vi "Inspect Address Pads.vi"(7 "Console Log in":refnum<class "Console Log.lvclass">, 8 "error in":errorcluster, 10 "Module Data In":T1={"TBM-TBM"={"Fiducial Image"={"Image Position"=refnum, "Image Reference"=refnum, "Field of View"={"x(mm)"=0.0, "y(mm)"=0.0}}, "Fiducials"=[]}, "TBM-HDI"={"Fiducial Image"={"Image Position"=refnum, "Image Reference"=refnum, "Field of View"={"x(mm)"=0.0, "y(mm)"=0.0}}, "Fiducials"=[]}, "Address Pads"={"Fiducial Image"={"Image Position"=refnum, "Image Reference"=refnum, "Field of View"={"x(mm)"=0.0, "y(mm)"=0.0}}, "Fiducials"=[]}, "HDI Bond Pad References"=[], "BBM Bond Pad References"=[], "HV-HDI"={"Fiducial Image"={"Image Position"=refnum, "Image Reference"=refnum, "Field of View"={"x(mm)"=0.0, "y(mm)"=0.0}}, "Selected Fiducial"={"Fiducial Image Coordinate"=refnum, "Fiducial Source"=enum."Pattern Recognition"}, "fiducial name"=""}, "HV-BBM"={"Fiducial Image"={"Image Position"=refnum, "Image Reference"=refnum, "Field of View"={"x(mm)"=0.0, "y(mm)"=0.0}}, "Selected Fiducial"={"Fiducial Image Coordinate"=refnum, "Fiducial Source"=enum."Pattern Recognition"}, "fiducial name"=""}, "Chuck"=0, "Slot"=0, "Potting Selection"={"HDI Bond Pads"=[TRUE, TRUE, TRUE, TRUE, TRUE, TRUE, TRUE, TRUE, TRUE, TRUE, TRUE, TRUE, TRUE, TRUE, TRUE, TRUE], "BBM Bond Pads"=[TRUE, TRUE, TRUE, TRUE, TRUE, TRUE, TRUE, TRUE, TRUE, TRUE, TRUE, TRUE, TRUE, TRUE, TRUE, TRUE], "TBM Inner"={"Top"=TRUE, "Left"=TRUE, "Bottom"=TRUE, "Right"=TRUE}, "TBM Outer"={"Top"=TRUE, "Left"=TRUE, "Bottom"=TRUE, "Right"=TRUE}, "Address Pads"={"Top"=TRUE, "Bottom"=TRUE}, "High Voltage"={"HDI"=TRUE, "BBM"=TRUE}}}, 11 "Potting Procedure in":refnum<class "Potting Procedure.lvclass">) -> (0 "error out":errorcluster, 2 "Module Data Out":T1={"TBM-TBM"={"Fiducial Image"={"Image Position"=refnum, "Image Reference"=refnum, "Field of View"={"x(mm)"=0.0, "y(mm)"=0.0}}, "Fiducials"=[]}, "TBM-HDI"={"Fiducial Image"={"Image Position"=refnum, "Image Reference"=refnum, "Field of View"={"x(mm)"=0.0, "y(mm)"=0.0}}, "Fiducials"=[]}, "Address Pads"={"Fiducial Image"={"Image Position"=refnum, "Image Reference"=refnum, "Field of View"={"x(mm)"=0.0, "y(mm)"=0.0}}, "Fiducials"=[]}, "HDI Bond Pad References"=[], "BBM Bond Pad References"=[], "HV-HDI"={"Fiducial Image"={"Image Position"=refnum, "Image Reference"=refnum, "Field of View"={"x(mm)"=0.0, "y(mm)"=0.0}}, "Selected Fiducial"={"Fiducial Image Coordinate"=refnum, "Fiducial Source"=enum."Pattern Recognition"}, "fiducial name"=""}, "HV-BBM"={"Fiducial Image"={"Image Position"=refnum, "Image Reference"=refnum, "Field of View"={"x(mm)"=0.0, "y(mm)"=0.0}}, "Selected Fiducial"={"Fiducial Image Coordinate"=refnum, "Fiducial Source"=enum."Pattern Recognition"}, "fiducial name"=""}, "Chuck"=0, "Slot"=0, "Potting Selection"={"HDI Bond Pads"=[TRUE, TRUE, TRUE, TRUE, TRUE, TRUE, TRUE, TRUE, TRUE, TRUE, TRUE, TRUE, TRUE, TRUE, TRUE, TRUE], "BBM Bond Pads"=[TRUE, TRUE, TRUE, TRUE, TRUE, TRUE, TRUE, TRUE, TRUE, TRUE, TRUE, TRUE, TRUE, TRUE, TRUE, TRUE], "TBM Inner"={"Top"=TRUE, "Left"=TRUE, "Bottom"=TRUE, "Right"=TRUE}, "TBM Outer"={"Top"=TRUE, "Left"=TRUE, "Bottom"=TRUE, "Right"=TRUE}, "Address Pads"={"Top"=TRUE, "Bottom"=TRUE}, "High Voltage"={"HDI"=TRUE, "BBM"=TRUE}}}, 3 "Potting Procedure out":refnum<class "Potting Procedure.lvclass">, 5 "Console Log out":refnum<class "Console Log.lvclass">)   [LabVIEW 2011, in "Potting Procedure.lvclass"]
uses:
  Potting Procedure.lvclass
  Application Utilities/Console Log/Console Log.lvclass
  Type Definitions/Inspect Modules - Module.ctl
  Shared Components/Vec3d Class/Vec3d Class.lvclass
  Shared Components/Utils/Type Definitions/Multi-Fiducial Image.ctl
  Shared Components/Utils/Type Definitions/Physical Image.ctl
  <vilib>/vision/Image Controls.llb/IMAQ Image.ctl
  Shared Components/Utils/Type Definitions/Fiducial with Source.ctl
  Shared Components/Utils/Type Definitions/Fiducial Image.ctl
  Shared Components/Config Manager Class/Type Definitions/Part Type.ctl
  Shared Components/Gantry Class/Gantry Class.lvclass
  Shared Components/WorkTable Class/WorkTable Class.lvclass
  Shared Components/Config Manager Class/Read Geometry Definition 3D.vi
  Shared Components/CameraTool Class/Take Area Image.vi
  Shared Components/CameraTool Class/CameraTool Class.lvclass
  Shared Components/Config Manager Class/Config Manager Class.lvclass
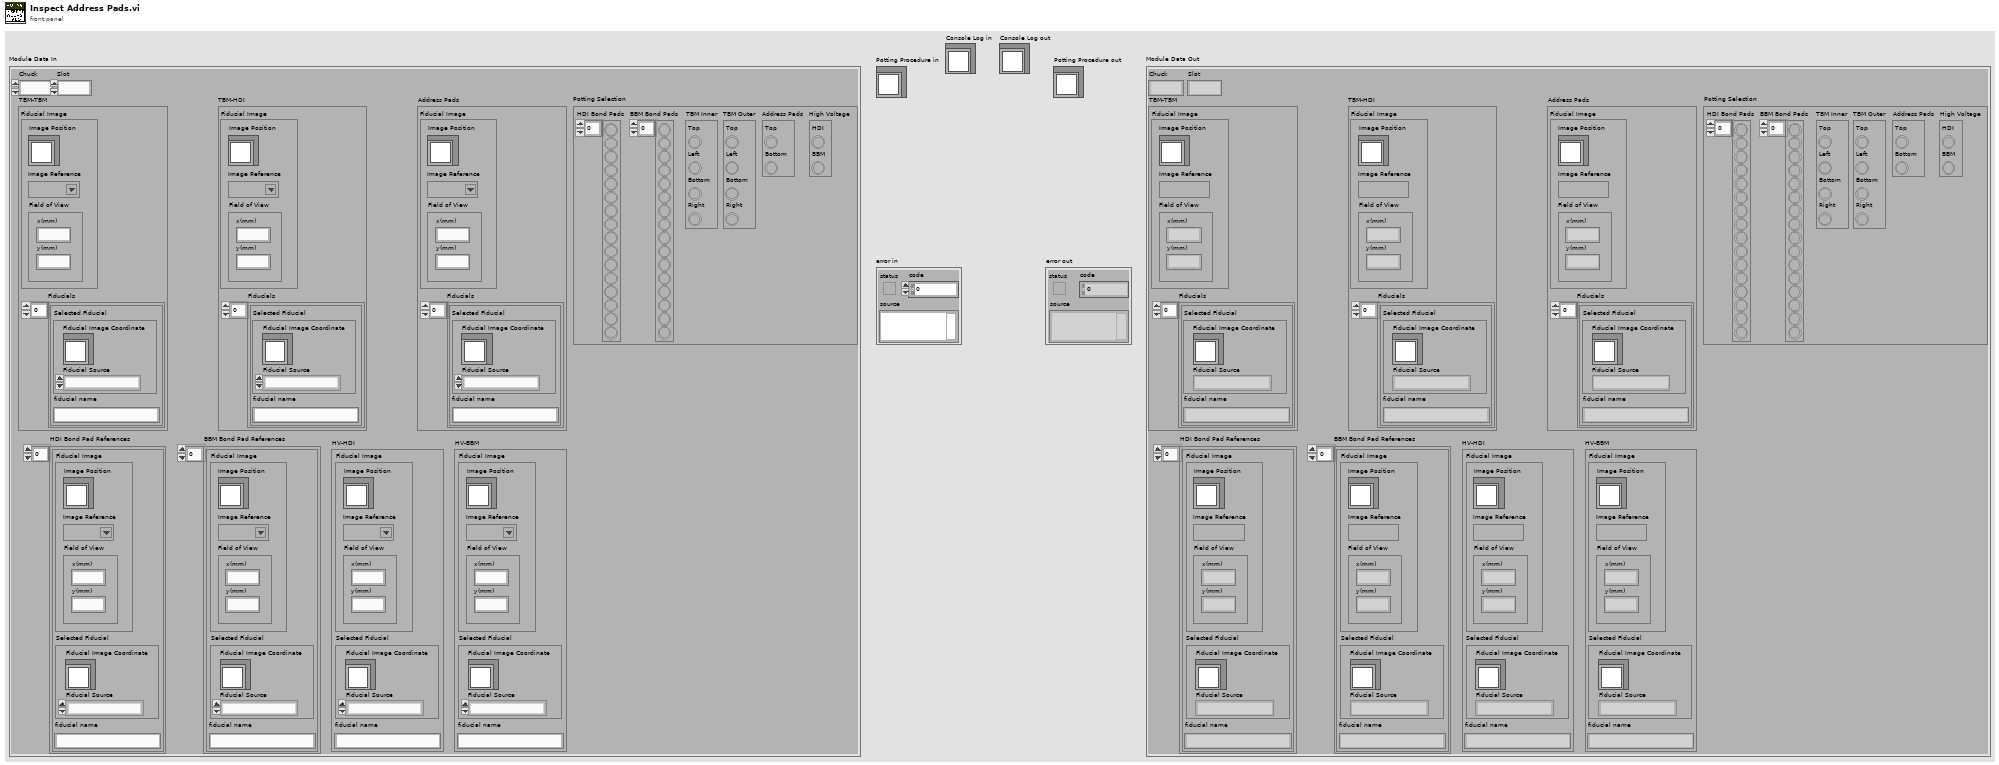
[diagram p1: front panel]
types:
  T1 = typedef "Inspect Modules - Module.ctl" = cluster{"TBM-TBM":T2, "TBM-HDI":T2, "Address Pads":T2, "HDI Bond Pad References":T6[], "BBM Bond Pad References":T6[], "HV-HDI":T6, "HV-BBM":T6, "Chuck":i32, "Slot":i32, "Potting Selection":cluster{"HDI Bond Pads":bool[], "BBM Bond Pads":bool[], "TBM Inner":cluster{"Top":bool, "Left":bool, "Bottom":bool, "Right":bool}, "TBM Outer":cluster{"Top":bool, "Left":bool, "Bottom":bool, "Right":bool}, "Address Pads":cluster{"Top":bool, "Bottom":bool}, "High Voltage":cluster{"HDI":bool, "BBM":bool}}}
  T2 = typedef "Multi-Fiducial Image.ctl" = cluster{"Fiducial Image":T3, "Fiducials":cluster{"Selected Fiducial":T5, "fiducial name":string}[]}
  T3 = typedef "Physical Image.ctl" = cluster{"Image Position":refnum<class "Vec3d Class.lvclass">, "Image Reference":T4, "Field of View":cluster{"x(mm)":dbl, "y(mm)":dbl}}
  T4 = typedef "IMAQ Image.ctl" = refnum<image>
  T5 = typedef "Fiducial with Source.ctl" = cluster{"Fiducial Image Coordinate":refnum<class "Vec3d Class.lvclass">, "Fiducial Source":enum16{"Pattern Recognition", "User", "Error", "Default"}}
  T6 = typedef "Fiducial Image.ctl" = cluster{"Fiducial Image":T3, "Selected Fiducial":T5, "fiducial name":string}
  T7 = enum16{"Pattern Recognition", "User", "Error", "Default"}
  T8 = cluster{"Selected Fiducial":T5, "fiducial name":string}
  T9 = typedef "Part Type.ctl" = enum16{"BBM", "HDI", "BARE HDI", "GLUERESERVOIR", "STAMP_1", "STAMP_2", "STAMP_3", "STAMP_4", "STAMP_5", "WEIGHT_1", "WEIGHT_2", "WEIGHT_3", "WEIGHT_4", "WEIGHT_5", "WEIGHT_6", "WEIGHT_7", "WEIGHT_8", "PICKER_TOOL", "GRABER_TOOL"}
  T10 = typedef "Worktable_Module Slot.ctl" = cluster{"Slot State":enum16{"Empty", "Bare HDI", "Unglued", "Stamped", "PartOnTop", "Weighted", "Unpotted", "Potted"}, "BBM Type":enum16{"None", "BBM", "GlassSlide"}, "HDI Type":enum16{"None", "HDI", "Polyimide"}, "Vacuum Channel":u8, "Location/Orientation BBM":T11, "Location/Orientation HDI":T11, "S/N":string}
  T11 = typedef "Position_Orientation.ctl" = cluster{"Center":refnum<class "Vec3d Class.lvclass">, "Orientation":refnum<class "Orient3d Class.lvclass">}
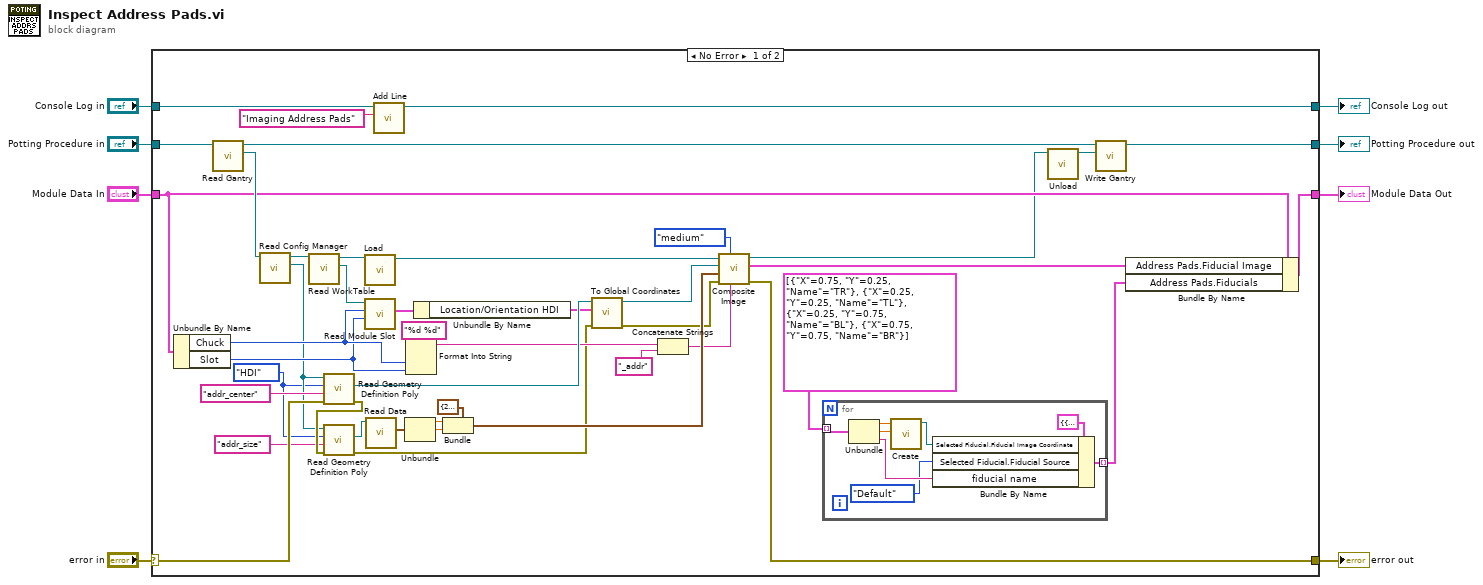
[diagram p0: block diagram]
diagram:
  n1 = case shown="No Error" "error in" {
    selector: "error in" -> [w49 w64]
    tunnel: [w16 w64] -> w7
    tunnel: [w22 w63] -> w8
    tunnel: "Potting Procedure in" -> [w52 w63]
    tunnel: "Module Data In" -> [w26 w62]
    tunnel: [w23 w62] -> w1
    tunnel: "Console Log in" -> [w14 w61]
    tunnel: [w13 w61] -> w3
    frame No Error {
      w10 = Part_Type."HDI" ("Part Type")
      n2 = Unbundle By Name(w26) -> ("Chuck"=w28:i32, "Slot"=w27:i32)
      n3 = call-dynamic "Read Gantry.vi"("Potting Procedure in"=w52) -> ("Gantry"=w50:refnum<class "Gantry Class.lvclass">, "Potting Procedure out"=w21:refnum<class "Potting Procedure.lvclass">)  [unwired: 8 in, 1 out]
      n4 = call-dynamic "Read Config Manager.vi"("Gantry in"=w50) -> ("Config Manager"=w11:refnum<class "Config Manager Class.lvclass">, "Gantry out"=w39:refnum<class "Gantry Class.lvclass">)  [unwired: 8 in, 1 out]
      n5 = call-dynamic "Read WorkTable.vi"("Gantry Class in"=w39) -> ("WorkTable Class.lvclass"=w37:refnum<class "WorkTable Class.lvclass">, "Gantry Class out"=w38:refnum<class "Gantry Class.lvclass">)  [unwired: 8 in, 1 out]
      n6 = call-poly "Read Geometry Definition Poly.vi"("error in"=w49, "Feature"="addr_center", "Part Type"=w10, "Config Manager in"=w11) -> ("error out"=w48:errorcluster, "Feature Coordinates"=w35:refnum<class "Vec3d Class.lvclass">)  [unwired: 5 in, 1 out]
      n7 = call-poly "Read Geometry Definition Poly.vi"("error in"=w48, "Feature"="addr_size", "Part Type"=w10, "Config Manager in"=w11) -> ("error out"=w19:errorcluster, "Feature Coordinates"=w45:refnum<class "Vec3d Class.lvclass">)  [unwired: 5 in, 1 out]
      n8 = call "Load.vi"("Gantry In"=w38) -> ("CameraTool out"=w51:refnum<class "CameraTool Class.lvclass">)  [unwired: 9 in, 1 out]
      n9 = call-dynamic "Read Module Slot.vi"("slot"=w27, "chuck"=w28, "WorkTable in"=w37) -> ("Module Slot"=w36:T10)  [unwired: 6 in, 2 out]
      n10 = call-dynamic "Read Data.vi"("Vec3d Class in"=w45) -> ("Data"=w44:cluster{"X":dbl, "Y":dbl, "Z":dbl})  [unwired: 8 in, 2 out]
      n11 = call "Add Line.vi"("String"="Imaging Address Pads", "Console Log in"=w14) -> ("Console Log out"=w13:refnum<class "Console Log.lvclass">)  [unwired: 8 in, 1 out]
      n12 = Unbundle(w44) -> ("X"=w43:dbl, "Y"=w42:dbl)  [unwired: 1 out]
      n13 = Format Into String(format string="%d %d", w28, w27) -> (resulting string=w30:string)  [unwired: 2 in, 1 out]
      n14 = Unbundle By Name(w36) -> ("Location/Orientation HDI"=w34:T11)
      n15 = Bundle(cluster=cluster{"Size-X(mm)":dbl, "Size-Y(mm)":dbl} {"Size-X(mm)"=20.0, "Size-Y(mm)"=20.0} ("Field of View"), "Size-X(mm)"=w43, "Size-Y(mm)"=w42) -> (w41:cluster{"Size-X(mm)":dbl, "Size-Y(mm)":dbl})
      n16 = call "To Global Coordinates.vi"("error in"=w19, "Center/Orientation"=w34, "Local Coordinates"=w35) -> ("error out"=w33:errorcluster, "Global Coordinates"=w17:refnum<class "Vec3d Class.lvclass">)  [unwired: 7 in]
      n17 = Concatenate Strings(w30, "_addr" ("string")) -> (w29:string)
      n18 = call-poly "Composite Image.vi"("Image Name"=w29, "Quality"=enum16{"perfect", "high", "medium", "low"}."medium", "error in"=w33, "Field of View"=w41, "Image Center"=w17, "CameraTool in"=w51) -> ("error out"=w16:errorcluster, "Physical Image"=w25:T3, "CameraTool out"=w18:refnum<class "CameraTool Class.lvclass">)  [unwired: 3 in]
      n19 = for {
        tunnel: cluster{"X":dbl, "Y":dbl, "Name":string}[] [{"X"=0.75, "Y"=0.25, "Name"="TR"}, {"X"=0.25, "Y"=0.25, "Name"="TL"}, {"X"=0.25, "Y"=0.75, "Name"="BL"}, {"X"=0.75, "Y"=0.75, "Name"="BR"}] -> [w59] mode=indexing
        tunnel: [w53] -> w15 mode=indexing
        n20 = Unbundle(w59) -> ("X"=w57:dbl, "Y"=w58:dbl, "Name"=w55:string)
        n21 = call "Create.vi"("Y"=w58, "X"=w57) -> ("Vec3d Class out"=w56:refnum<class "Vec3d Class.lvclass">)  [unwired: 8 in, 1 out]
        n22 = Bundle By Name(cluster=T8 {"Selected Fiducial"={"Fiducial Image Coordinate"=refnum, "Fiducial Source"=enum."Pattern Recognition"}, "fiducial name"=""} ("Fiducial"), "Selected Fiducial.Fiducial Image Coordinate"=w56, "Selected Fiducial.Fiducial Source"=T7."Default", "fiducial name"=w55) -> (w53:T8)
      }
      n23 = call "Unload.vi"("CameraTool in"=w18) -> ("Gantry out"=w20:refnum<class "Gantry Class.lvclass">)  [unwired: 9 in, 1 out]
      n24 = call-dynamic "Write Gantry.vi"("Gantry"=w20, "Potting Procedure in"=w21) -> ("Potting Procedure out"=w22:refnum<class "Potting Procedure.lvclass">)  [unwired: 8 in, 1 out]
      n25 = Bundle By Name(cluster=w26, "Address Pads.Fiducial Image"=w25, "Address Pads.Fiducials"=w15) -> (w23:T1)
    }
    frame Error {
    }
  }
  "error out" <- w7
  "Potting Procedure out" <- w8
  "Console Log out" <- w3
  "Module Data Out" <- w1
